vi "氨氮总氮总磷质控流程.vi"(8 "总氮":bool, 9 "总磷":bool, 10 "氨氮":bool, 11 "队列输入":refnum<queue>) -> (3 "布尔":bool)   [LabVIEW 2016, in "质控单元.lvlib"]
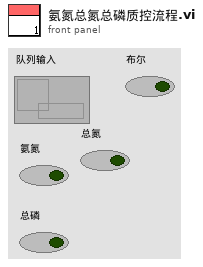
[diagram p1: front panel]
types:
  T1 = enum16{"待机", "启动氨氮水样", "氨氮测量中", "启动氨氮加标", "启动氨氮加标回收", "氨氮加标回收测量中", "启动总氮水样", "总氮测量中", "启动总氮加标", "启动总氮加标回收", "总氮加标回收测量中", "启动总磷水样", "总磷水样测量中", "启动总磷加标", "启动总磷加标回收", "总磷加标回收测量中", "结束"}
  T2 = cluster{"站号":u16, "量程切换":enum32{"H", "L", "AUTO"}, "控制命令":enum16{"启动测量", "标样核查", "零点核查", "跨度核查", "空白测试", "平行样测试", "加标回收", "空白校准", "标样校准", "初始化（清洗）", "停止测试", "仪器重启", "校时", "模式设置", "测量间隔设置"}, "模式设置":enum16{"待机", "连续模式", "周期模式", "定点模式", "受控模式", "手动模式"}, "测量间隔":u16}
  T3 = cluster{"时间标识":timestamp, "设备":string, "日志信息":string}
  T4 = cluster{"系统时间":timestamp, "工作状态":enum16{"空闲", "水样测试", "标样核查", "零点核查", "跨度核查", "空白测试", "平行样测试", "加标回收", "空白校准", "标样校准", "初始化（清洗）"}, "测量模式":enum16{"待机", "连续模式", "周期模式", "定点模式", "受控模式", "手动模式"}, "告警代码":enum16{"无告警", "缺试剂告警", "缺水样告警", "缺蒸馏水告警", "缺标液告警", "仪表漏液告警", "标定异常告警", "超量程告警", "加热异常", "低试剂预警", "超上限告警", "超下限告警", "仪表内部其他异常", "滴定异常告警", "电极异常告警", "量程切换告警", "参数设置告警", "PH电极电位异常", "电导率电极异常", "浊度光度异常", "溶解氧电极异常", "溶解氧光强异常", "温度异常告警", "PH异常告警", "溶解氧异常告警", "电导率异常告警", "浊度异常告警", "叶绿素异常告警", "藻密度异常告警", "蓝绿藻异常告警", "ORP异常告警", "氨氮异常告警", "清洁刷异常告警", "SD卡异常告警", "蓝牙异常告警", "Wifi异常告警", "流程异常告警"}, "故障代码":enum16{"无故障", "电机故障", "温度故障", "通讯故障", "滴定故障"}, "日志代码":u16, "软件版本":u16, "F0":sgl, "F1":sgl, "F2":sgl, "F3":sgl, "T":sgl, "H":sgl, "id":u16, "flowid":u16, "量程":u16}
  T5 = enum16{"空闲", "水样测试", "标样核查", "零点核查", "跨度核查", "空白测试", "平行样测试", "加标回收", "空白校准", "标样校准", "初始化（清洗）"}
  T6 = cluster{"因子编码":u32, "单位":u16, "标样参考值":sgl, "水样数据时间":timestamp, "水样实测值":sgl, "水样数据标识":string, "标样数据时间":timestamp, "标样实测值":sgl, "标样数据标识":string, "空白数据时间":timestamp, "空白实测值":sgl, "空白数据标识":string, "零点核查数据时间":timestamp, "零点核查实测值":sgl, "零点核查数据标识":string, "跨度核查数据时间":timestamp, "跨度核查实测值":sgl, "跨度核查数据标识":string, "加标回收数据时间":timestamp, "加标回收实测值":sgl, "加标回收数据标识":string, "平行样数据时间":timestamp, "平行样实测值":sgl, "平行样数据标识":string, "F0":sgl, "F1":sgl, "F2":sgl, "F3":sgl, "F4":sgl, "F5":sgl, "F6":sgl, "F7":sgl, "温度":sgl, "湿度":sgl, "X值":sgl}
  T7 = cluster{"量程":dbl, "检出限":dbl, "加标前水样浓度":dbl, "加标后水样浓度":dbl, "加标水杯定容体积":dbl, "加标母液浓度":dbl, "加标体积":dbl, "加标回收率":dbl}
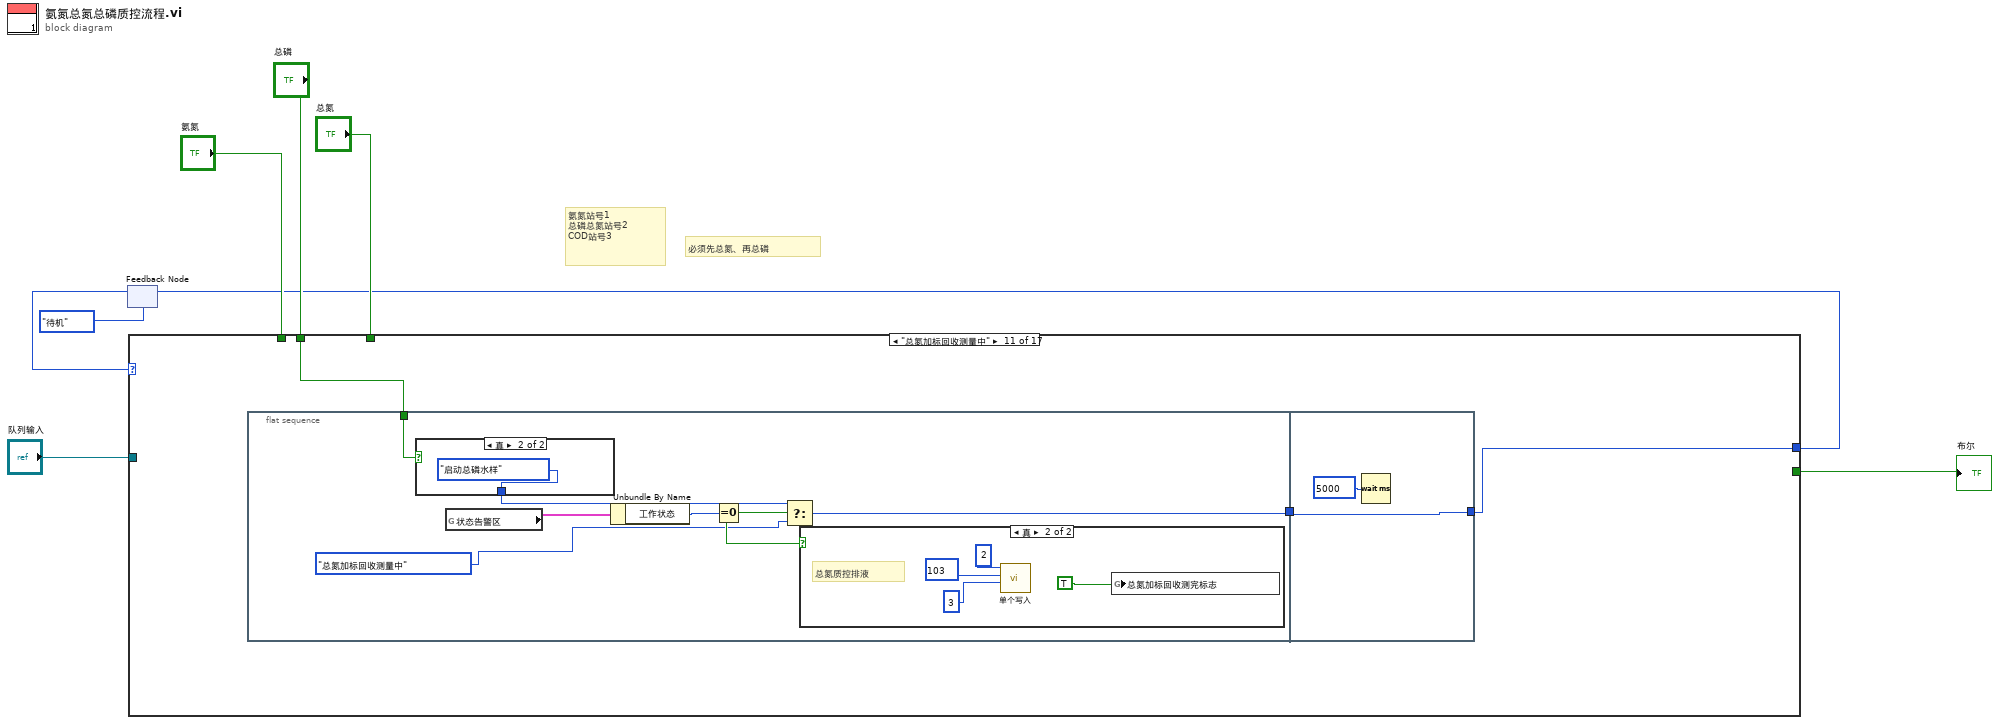
[diagram p0: block diagram]
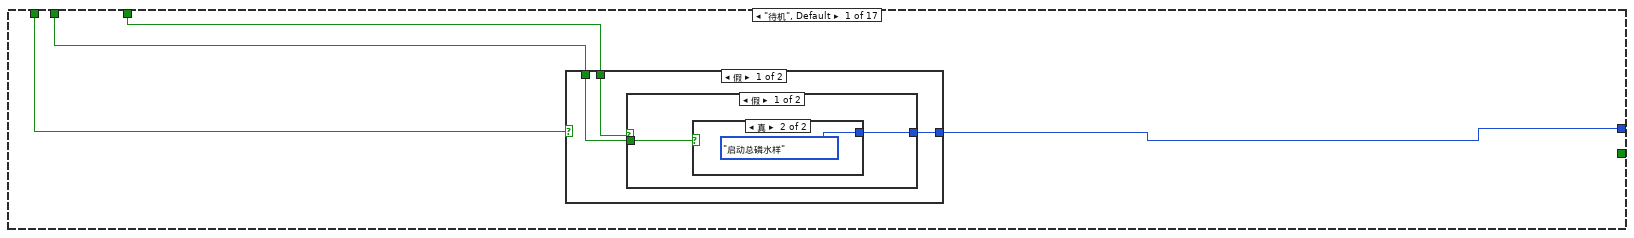
[diagram p2: hidden frame]
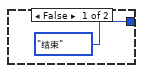
[diagram p3: hidden frame]
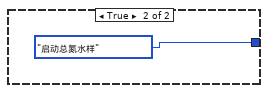
[diagram p4: hidden frame]
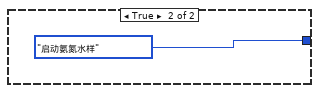
[diagram p5: hidden frame]
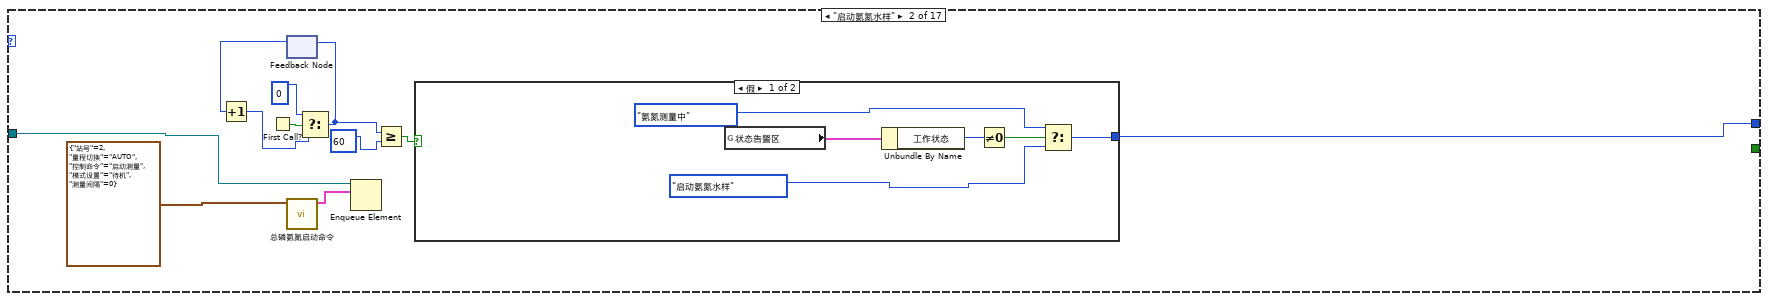
[diagram p6: hidden frame]
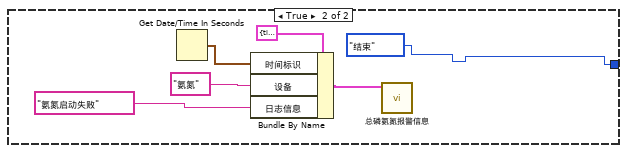
[diagram p7: hidden frame]
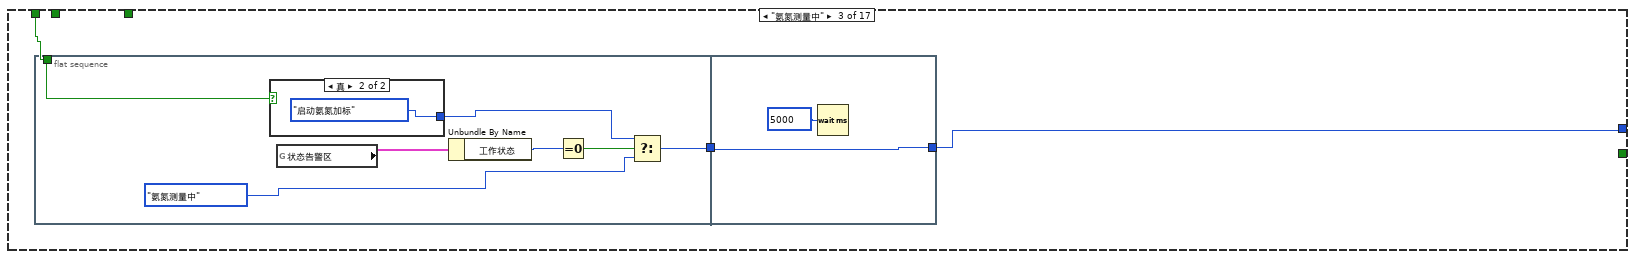
[diagram p8: hidden frame]
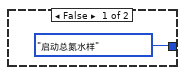
[diagram p9: hidden frame]
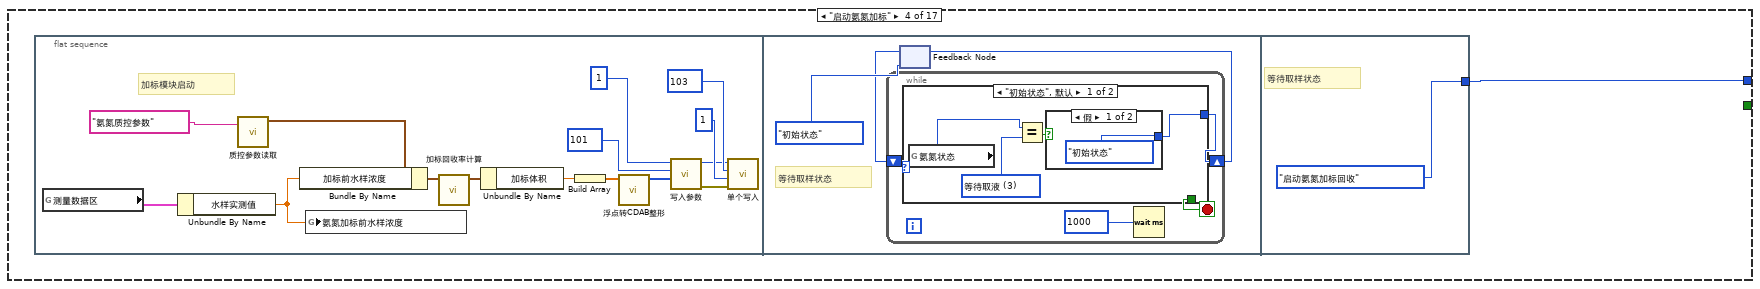
[diagram p10: hidden frame]
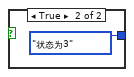
[diagram p11: hidden frame]
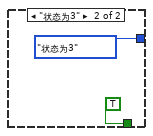
[diagram p12: hidden frame]
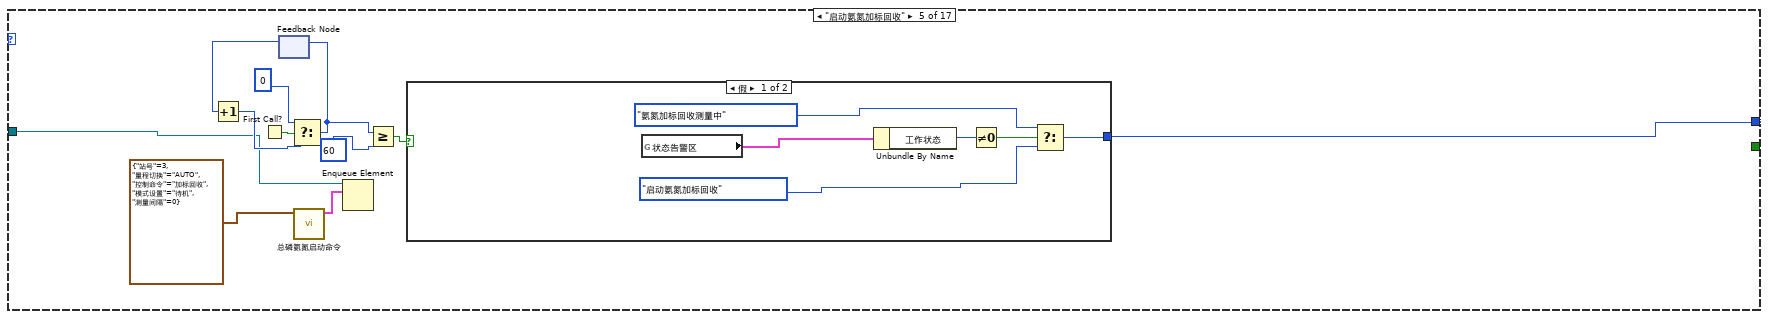
[diagram p13: hidden frame]
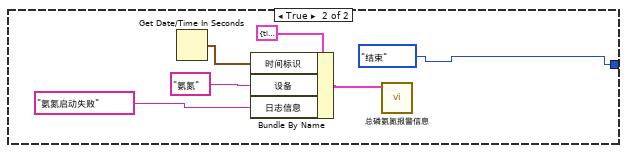
[diagram p14: hidden frame]
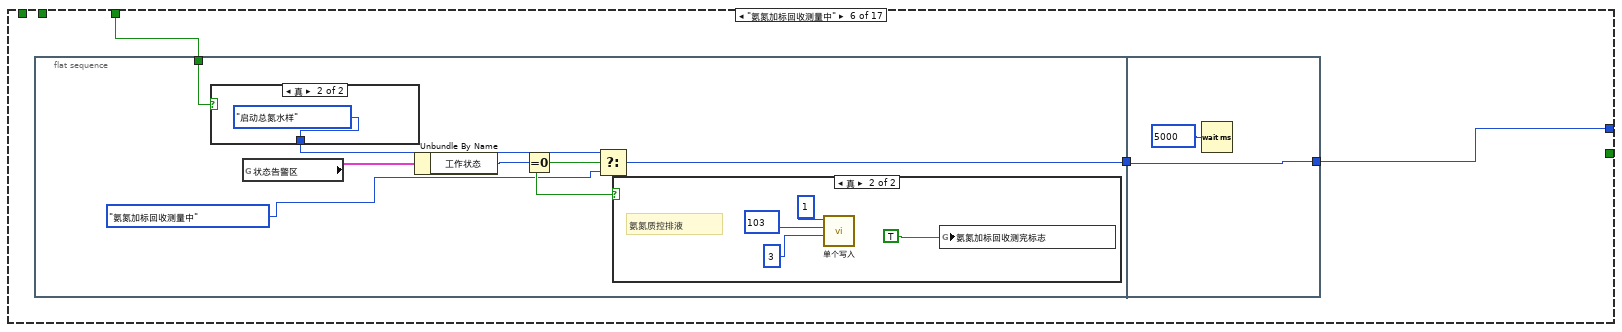
[diagram p15: hidden frame]
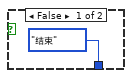
[diagram p16: hidden frame]
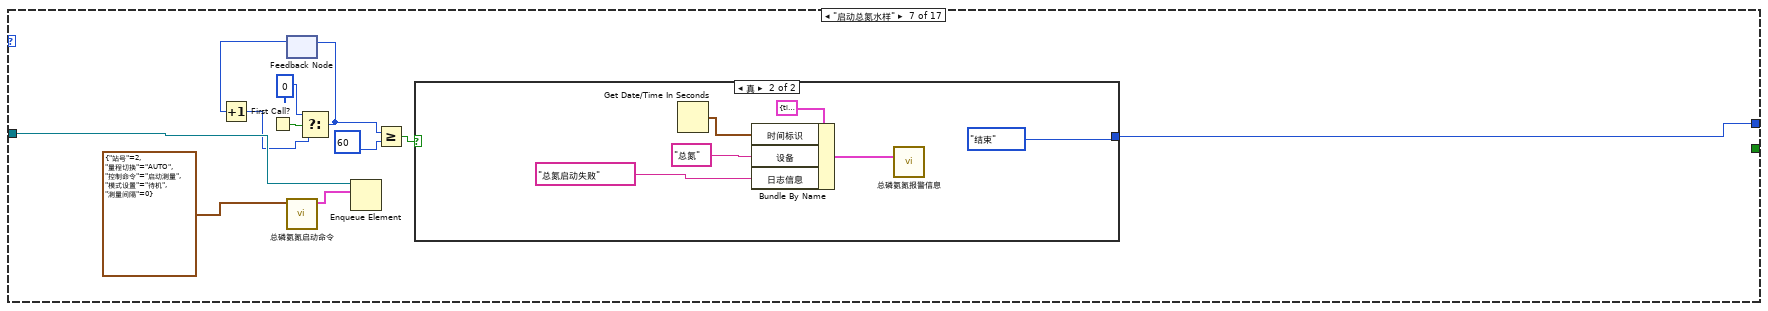
[diagram p18: hidden frame]
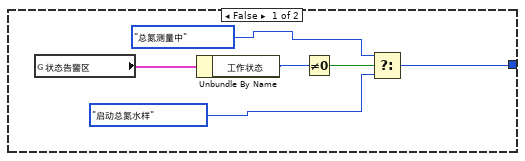
[diagram p19: hidden frame]
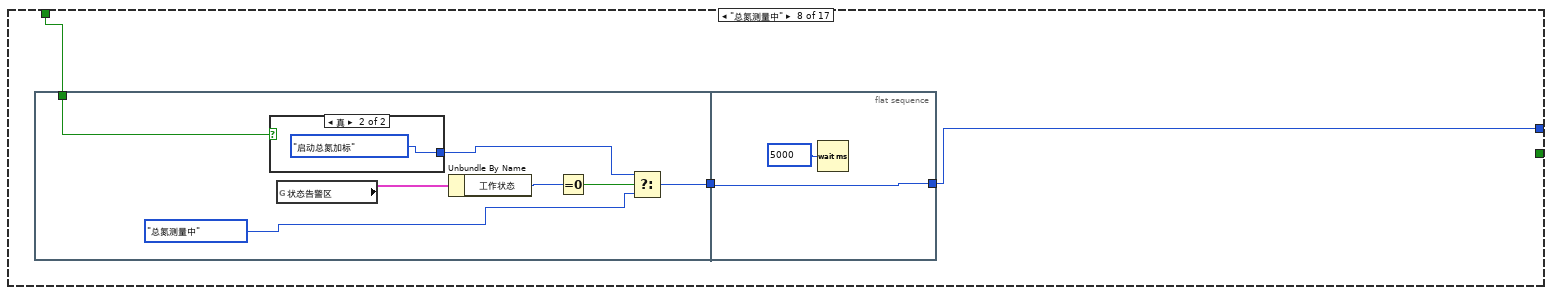
[diagram p20: hidden frame]
diagram:
  # "氨氮站号1   \n总磷总氮站号2\nCOD站号3"
  # "必须先总氮、再总磷"
  n1 = feedback #1(T1."待机") -> (w3:T1)
  n2 = case shown="\"总氮加标回收测量中\"" w3 {
    tunnel: [w12 w31 w47 w59 w92 w113 w140 w154 w168 w199 w222 w249 w265 w277 w309 w331 T1."结束"] -> w1
    tunnel: "队列输入" -> [_ w32 _ _ w93 _ w141 _ _ w202 _ w250 _ _ w310 _ _]
    tunnel: [_ _ _ _ _ _ _ _ _ _ _ _ _ _ _ _ TRUE] -> w6
    tunnel: "总磷" -> [w10 _ _ _ _ _ _ _ _ _ w223 _ w263 _ _ _ _]
    tunnel: "氨氮" -> [w11 _ w45 _ _ _ _ _ _ _ _ _ _ _ _ _ _]
    tunnel: "总氮" -> [w9 _ _ _ _ w114 _ w155 _ _ _ _ _ _ _ _ _]
    frame "待机", Default {
      n3 = case shown="假" w11 {
        tunnel: [w14 T1."启动氨氮水样"] -> w12
        tunnel: w10 -> [w15 _]
        tunnel: w9 -> [w13 _]
        frame False {
          n4 = case shown="假" w13 {
            tunnel: w15 -> [w16 _]
            tunnel: [w17 T1."启动总氮水样"] -> w14
            frame False {
              n5 = case shown="真" w16 {
                tunnel: [T1."结束" T1."启动总磷水样"] -> w17
                frame False {
                }
                frame True {
                }
              }
            }
            frame True {
            }
          }
        }
        frame True {
        }
      }
    }
    frame "启动氨氮水样" {
      n6 = First Call?() -> (First Call?: T/F=w29:bool)
      n7 = feedback #2() -> (w28:i32)  [unwired: 1 in]
      n8 = Increment(x=w28) -> (x+1=w27:i32)
      n9 = call "总磷氨氮启动命令.vi"("参数"=T2 {"站号"=2, "量程切换"=enum."AUTO", "控制命令"=enum."启动测量", "模式设置"=enum."待机", "测量间隔"=0}) -> ("启动命令"=w23:cluster{"命令":string, "data":variant})  [unwired: 10 in]
      n10 = Select(t=0, s=w29, f=w27) -> (s? t:f=w26:i32)
      n11 = feedback-in #2(w26) -> ()
      n12 = Enqueue Element(queue=w32, element=w23) -> ()  [unwired: 2 in, 3 out]
      n13 = Greater Or Equal?(x=w26, y=60) -> (x >= y?=w24:bool)
      n14 = case shown="假" w24 {
        tunnel: [w35 T1."结束"] -> w31
        frame False {
          n15 = global read "VAR总磷氨氮全局变量.vi" "状态告警区"() -> (w38:T4)
          n16 = Unbundle By Name(w38) -> ("工作状态"=w37:T5)
          n17 = Not Equal To 0?(x=w37) -> (x != 0?=w36:bool)
          n18 = Select(t=T1."氨氮测量中", s=w36, f=T1."启动氨氮水样") -> (s? t:f=w35:T1)
        }
        frame True {
          n19 = Get Date/Time In Seconds() -> (seconds since 1Jan1904=w44:timestamp)
          n20 = Bundle By Name(cluster=T3 {"时间标识"=timestamp(0 s since 1904-01-01), "设备"="", "日志信息"=""} ("data in"), "时间标识"=w44, "设备"="氨氮", "日志信息"="氨氮启动失败") -> (w40:T3)
          n21 = call "总磷氨氮报警信息.vi"("data in"=w40) -> ()  [unwired: 11 in]
        }
      }
    }
    frame "氨氮测量中" {
      n22 = flat-sequence {
        tunnel: [w52] -> w46
        tunnel: w45 -> [w49]
        tunnel: [w58] -> w47
        tunnel: w46 -> [w58]
        frame #0 {
          n23 = case shown="真" w49 {
            tunnel: [T1."启动总氮水样" T1."启动氨氮加标"] -> w50
            frame False {
            }
            frame True {
            }
          }
          n24 = global read "VAR总磷氨氮全局变量.vi" "状态告警区"() -> (w53:T4)
          n25 = Unbundle By Name(w53) -> ("工作状态"=w54:T5)
          n26 = Equal To 0?(x=w54) -> (x = 0?=w51:bool)
          n27 = Select(t=w50, s=w51, f=T1."氨氮测量中") -> (s? t:f=w52:T1)
        }
        frame #1 {
          n28 = Wait (ms)(milliseconds to wait=u32 5000 ("等待时间（毫秒）")) -> ()  [unwired: 1 out]
        }
      }
    }
    frame "启动氨氮加标" {
      n29 = flat-sequence {
        tunnel: [T1."启动氨氮加标回收"] -> w59
        frame #0 {
          w63 = u16 1 ("value")
          # "加标模块启动"
          n30 = global read "VAR总磷氨氮全局变量.vi" "测量数据区"() -> (w61:T6)
          n31 = Unbundle By Name(w61) -> ("水样实测值"=w60:sgl)
          n32 = call "质控参数读取.vi"("section"="氨氮质控参数") -> ("参数"=w71:T7)  [unwired: 9 in, 1 out]
          n33 = Bundle By Name(cluster=w71, "加标前水样浓度"=w60) -> (w72:T7)
          n34 = global write "水样浓度全局.vi" "氨氮加标前水样浓度"(w60) -> ()
          n35 = call "加标回收率计算.vi"("参数"=w72) -> ("参数 out"=w70:T7)  [unwired: 10 in]
          n36 = Unbundle By Name(w70) -> ("加标体积"=w62:dbl)
          n37 = Build Array(w62) -> (w69:dbl[])
          n38 = call "浮点转CDAB整形.vi"("浮点数"=w69) -> ("CDAB整形输出"=w64:u16[])  [unwired: 10 in]
          n39 = call "写入参数.vi"("values"=w64, "starting address"=u16 101, "Slave ID"=w63) -> ("error out"=w68:errorcluster)  [unwired: 8 in]
          n40 = call "单个写入.vi"("Error in"=w68, "value"=u16 1, "address"=u16 103, "Slave ID"=w63) -> ()  [unwired: 7 in, 1 out]
        }
        frame #1 {
          # "等待取样状态"
          n41 = feedback #3(enum16{"初始状态", "状态为3"}."初始状态") -> (w75:enum16{"初始状态", "状态为3"})
          n42 = while {
            shift-right: [w79] -> w74
            shift-left: w75 -> [w80]
            stop <- w78 stop-if-true
            n43 = case shown="\"初始状态\", 默认" w80 {
              tunnel: [w82 enum16{"初始状态", "状态为3"}."状态为3"] -> w79
              tunnel: [_ TRUE] -> w78
              frame "初始状态", Default {
                w81 = u16 3 items=["待机", "润洗", "进样", "等待取液", "排液"] ("氨氮状态")
                n44 = global read "氨氮加标回收状态全局变量.vi" "氨氮状态"() -> (w84:u16)
                n45 = Equal?(x=w84, y=w81) -> (x = y?=w83:bool)
                n46 = case shown="假" w83 {
                  tunnel: [enum16{"初始状态", "状态为3"}."初始状态" enum16{"初始状态", "状态为3"}."状态为3"] -> w82
                  frame False {
                  }
                  frame True {
                  }
                }
              }
              frame "状态为3" {
              }
            }
            n47 = Wait (ms)(milliseconds to wait=u32 1000 ("等待时间（毫秒）")) -> ()  [unwired: 1 out]
          }
          n48 = feedback-in #3(w74) -> ()
        }
        frame #2 {
          # "等待取样状态"
        }
      }
    }
    frame "启动氨氮加标回收" {
      n49 = First Call?() -> (First Call?: T/F=w99:bool)
      n50 = feedback #4() -> (w98:i32)  [unwired: 1 in]
      n51 = Increment(x=w98) -> (x+1=w97:i32)
      n52 = Select(t=0, s=w99, f=w97) -> (s? t:f=w96:i32)
      n53 = feedback-in #4(w96) -> ()
      n54 = call "总磷氨氮启动命令.vi"("参数"=T2 {"站号"=3, "量程切换"=enum."AUTO", "控制命令"=enum."加标回收", "模式设置"=enum."待机", "测量间隔"=0}) -> ("启动命令"=w91:cluster{"命令":string, "data":variant})  [unwired: 10 in]
      n55 = Enqueue Element(queue=w93, element=w91) -> ()  [unwired: 2 in, 3 out]
      n56 = Greater Or Equal?(x=w96, y=60) -> (x >= y?=w94:bool)
      n57 = case shown="假" w94 {
        tunnel: [w103 T1."结束"] -> w92
        frame False {
          n58 = global read "VAR总磷氨氮全局变量.vi" "状态告警区"() -> (w106:T4)
          n59 = Unbundle By Name(w106) -> ("工作状态"=w105:T5)
          n60 = Not Equal To 0?(x=w105) -> (x != 0?=w104:bool)
          n61 = Select(t=T1."氨氮加标回收测量中", s=w104, f=T1."启动氨氮加标回收") -> (s? t:f=w103:T1)
        }
        frame True {
          n62 = Get Date/Time In Seconds() -> (seconds since 1Jan1904=w112:timestamp)
          n63 = Bundle By Name(cluster=T3 {"时间标识"=timestamp(0 s since 1904-01-01), "设备"="", "日志信息"=""} ("data in"), "时间标识"=w112, "设备"="氨氮", "日志信息"="氨氮启动失败") -> (w108:T3)
          n64 = call "总磷氨氮报警信息.vi"("data in"=w108) -> ()  [unwired: 11 in]
        }
      }
    }
    frame "氨氮加标回收测量中" {
      n65 = flat-sequence {
        tunnel: [w120] -> w115
        tunnel: w114 -> [w117]
        tunnel: [w130] -> w113
        tunnel: w115 -> [w130]
        frame #0 {
          n66 = case shown="真" w117 {
            tunnel: [T1."结束" T1."启动总氮水样"] -> w119
            frame False {
            }
            frame True {
            }
          }
          n67 = global read "VAR总磷氨氮全局变量.vi" "状态告警区"() -> (w121:T4)
          n68 = Unbundle By Name(w121) -> ("工作状态"=w122:T5)
          n69 = Equal To 0?(x=w122) -> (x = 0?=w118:bool)
          n70 = Select(t=w119, s=w118, f=T1."氨氮加标回收测量中") -> (s? t:f=w120:T1)
          n71 = case shown="真" w118 {
            frame False {
            }
            frame True {
              # "氨氮质控排液"
              n72 = call "单个写入.vi"("value"=u16 3, "address"=u16 103, "Slave ID"=u8 1) -> ()  [unwired: 8 in, 1 out]
              n73 = global write "质控测完标志全局 1.vi" "氨氮加标回收测完标志"(TRUE) -> ()
            }
          }
        }
        frame #1 {
          n74 = Wait (ms)(milliseconds to wait=u32 5000 ("等待时间（毫秒）")) -> ()  [unwired: 1 out]
        }
      }
    }
    frame "启动总氮水样" {
      n75 = First Call?() -> (First Call?: T/F=w138:bool)
      n76 = feedback #5() -> (w137:i32)  [unwired: 1 in]
      n77 = Increment(x=w137) -> (x+1=w136:i32)
      n78 = call "总磷氨氮启动命令.vi"("参数"=T2 {"站号"=2, "量程切换"=enum."AUTO", "控制命令"=enum."启动测量", "模式设置"=enum."待机", "测量间隔"=0}) -> ("启动命令"=w132:cluster{"命令":string, "data":variant})  [unwired: 10 in]
      n79 = Select(t=0, s=w138, f=w136) -> (s? t:f=w135:i32)
      n80 = feedback-in #5(w135) -> ()
      n81 = Enqueue Element(queue=w141, element=w132) -> ()  [unwired: 2 in, 3 out]
      n82 = Greater Or Equal?(x=w135, y=60) -> (x >= y?=w133:bool)
      n83 = case shown="真" w133 {
        tunnel: [w144 T1."结束"] -> w140
        frame False {
          n84 = global read "VAR总磷氨氮全局变量.vi" "状态告警区"() -> (w145:T4)
          n85 = Unbundle By Name(w145) -> ("工作状态"=w146:T5)
          n86 = Not Equal To 0?(x=w146) -> (x != 0?=w147:bool)
          n87 = Select(t=T1."总氮测量中", s=w147, f=T1."启动总氮水样") -> (s? t:f=w144:T1)
        }
        frame True {
          n88 = Get Date/Time In Seconds() -> (seconds since 1Jan1904=w153:timestamp)
          n89 = Bundle By Name(cluster=T3 {"时间标识"=timestamp(0 s since 1904-01-01), "设备"="", "日志信息"=""} ("data in"), "时间标识"=w153, "设备"="总氮", "日志信息"="总氮启动失败") -> (w149:T3)
          n90 = call "总磷氨氮报警信息.vi"("data in"=w149) -> ()  [unwired: 11 in]
        }
      }
    }
    frame "总氮测量中" {
      n91 = flat-sequence {
        tunnel: [w161] -> w156
        tunnel: w155 -> [w158]
        tunnel: [w167] -> w154
        tunnel: w156 -> [w167]
        frame #0 {
          n92 = case shown="真" w158 {
            tunnel: [T1."启动总磷水样" T1."启动总氮加标"] -> w159
            frame False {
            }
            frame True {
            }
          }
          n93 = global read "VAR总磷氨氮全局变量.vi" "状态告警区"() -> (w162:T4)
          n94 = Unbundle By Name(w162) -> ("工作状态"=w163:T5)
          n95 = Equal To 0?(x=w163) -> (x = 0?=w160:bool)
          n96 = Select(t=w159, s=w160, f=T1."总氮测量中") -> (s? t:f=w161:T1)
        }
        frame #1 {
          n97 = Wait (ms)(milliseconds to wait=u32 5000 ("等待时间（毫秒）")) -> ()  [unwired: 1 out]
        }
      }
    }
    frame "启动总氮加标" {
      n98 = flat-sequence {
        tunnel: [T1."启动总氮加标回收"] -> w168
        frame #0 {
          w173 = u16 2 ("value")
          # "加标模块启动"
          n99 = global read "VAR总磷氨氮全局变量.vi" "测量数据区"() -> (w171:T6)
          n100 = Unbundle By Name(w171) -> ("水样实测值"=w169:sgl)
          n101 = call "质控参数读取.vi"("section"="总氮质控参数") -> ("参数"=w170:T7)  [unwired: 9 in, 1 out]
          n102 = Bundle By Name(cluster=w170, "加标前水样浓度"=w169) -> (w181:T7)
          n103 = global write "水样浓度全局.vi" "总氮加标前水样浓度"(w169) -> ()
          n104 = call "加标回收率计算.vi"("参数"=w181) -> ("参数 out"=w180:T7)  [unwired: 10 in]
          n105 = Unbundle By Name(w180) -> ("加标体积"=w172:dbl)
          n106 = Build Array(w172) -> (w179:dbl[])
          n107 = call "浮点转CDAB整形.vi"("浮点数"=w179) -> ("CDAB整形输出"=w174:u16[])  [unwired: 10 in]
          n108 = call "写入参数.vi"("values"=w174, "starting address"=u16 101, "Slave ID"=w173) -> ("error out"=w178:errorcluster)  [unwired: 8 in]
          n109 = call "单个写入.vi"("Error in"=w178, "value"=u16 2, "address"=u16 103, "Slave ID"=w173) -> ()  [unwired: 7 in, 1 out]
        }
        frame #1 {
          # "等待取样状态"
          n110 = feedback #6(enum16{"初始状态", "状态为3"}."初始状态") -> (w184:enum16{"初始状态", "状态为3"})
          n111 = while {
            shift-right: [w188] -> w183
            shift-left: w184 -> [w189]
            stop <- w187 stop-if-true
            n112 = case shown="\"状态为3\"" w189 {
              tunnel: [w190 enum16{"初始状态", "状态为3"}."状态为3"] -> w188
              tunnel: [_ TRUE] -> w187
              frame "初始状态", Default {
                n113 = global read "氨氮加标回收状态全局变量.vi" "总磷状态"() -> (w192:u16)
                n114 = Equal?(x=w192, y=u16 3) -> (x = y?=w191:bool)
                n115 = case shown="真" w191 {
                  tunnel: [enum16{"初始状态", "状态为3"}."初始状态" enum16{"初始状态", "状态为3"}."状态为3"] -> w190
                  frame False {
                  }
                  frame True {
                  }
                }
              }
              frame "状态为3" {
              }
            }
            n116 = Wait (ms)(milliseconds to wait=u32 1000 ("等待时间（毫秒）")) -> ()  [unwired: 1 out]
          }
          n117 = feedback-in #6(w183) -> ()
        }
        frame #2 {
          # "等待取样状态"
        }
      }
    }
    frame "启动总氮加标回收" {
      n118 = First Call?() -> (First Call?: T/F=w208:bool)
      n119 = feedback #7() -> (w207:i32)  [unwired: 1 in]
      n120 = Increment(x=w207) -> (x+1=w206:i32)
      n121 = call "总磷氨氮启动命令.vi"("参数"=T2 {"站号"=2, "量程切换"=enum."AUTO", "控制命令"=enum."加标回收", "模式设置"=enum."待机", "测量间隔"=0}) -> ("启动命令"=w200:cluster{"命令":string, "data":variant})  [unwired: 10 in]
      n122 = Select(t=0, s=w208, f=w206) -> (s? t:f=w205:i32)
      n123 = feedback-in #7(w205) -> ()
      n124 = Enqueue Element(queue=w202, element=w200) -> ()  [unwired: 2 in, 3 out]
      n125 = Greater Or Equal?(x=w205, y=60) -> (x >= y?=w203:bool)
      n126 = case shown="假" w203 {
        tunnel: [w212 T1."结束"] -> w199
        frame False {
          n127 = global read "VAR总磷氨氮全局变量.vi" "状态告警区"() -> (w215:T4)
          n128 = Unbundle By Name(w215) -> ("工作状态"=w214:T5)
          n129 = Not Equal To 0?(x=w214) -> (x != 0?=w213:bool)
          n130 = Select(t=T1."总氮加标回收测量中", s=w213, f=T1."启动总氮加标回收") -> (s? t:f=w212:T1)
        }
        frame True {
          n131 = Get Date/Time In Seconds() -> (seconds since 1Jan1904=w221:timestamp)
          n132 = Bundle By Name(cluster=T3 {"时间标识"=timestamp(0 s since 1904-01-01), "设备"="", "日志信息"=""} ("data in"), "时间标识"=w221, "设备"="氨氮", "日志信息"="氨氮启动失败") -> (w217:T3)
          n133 = call "总磷氨氮报警信息.vi"("data in"=w217) -> ()  [unwired: 11 in]
        }
      }
    }
    frame "总氮加标回收测量中" {
      n134 = flat-sequence {
        tunnel: [w229] -> w224
        tunnel: w223 -> [w226]
        tunnel: [w239] -> w222
        tunnel: w224 -> [w239]
        frame #0 {
          n135 = case shown="真" w226 {
            tunnel: [T1."结束" T1."启动总磷水样"] -> w228
            frame False {
            }
            frame True {
            }
          }
          n136 = global read "VAR总磷氨氮全局变量.vi" "状态告警区"() -> (w230:T4)
          n137 = Unbundle By Name(w230) -> ("工作状态"=w231:T5)
          n138 = Equal To 0?(x=w231) -> (x = 0?=w227:bool)
          n139 = Select(t=w228, s=w227, f=T1."总氮加标回收测量中") -> (s? t:f=w229:T1)
          n140 = case shown="真" w227 {
            frame False {
            }
            frame True {
              # "总氮质控排液"
              n141 = call "单个写入.vi"("value"=u16 3, "address"=u16 103, "Slave ID"=u8 2) -> ()  [unwired: 8 in, 1 out]
              n142 = global write "质控测完标志全局 1.vi" "总氮加标回收测完标志"(TRUE) -> ()
            }
          }
        }
        frame #1 {
          n143 = Wait (ms)(milliseconds to wait=u32 5000 ("等待时间（毫秒）")) -> ()  [unwired: 1 out]
        }
      }
    }
    frame "启动总磷水样" {
      n144 = First Call?() -> (First Call?: T/F=w247:bool)
      n145 = feedback #8() -> (w246:i32)  [unwired: 1 in]
      n146 = Increment(x=w246) -> (x+1=w245:i32)
      n147 = call "总磷氨氮启动命令.vi"("参数"=T2 {"站号"=1, "量程切换"=enum."AUTO", "控制命令"=enum."启动测量", "模式设置"=enum."待机", "测量间隔"=0}) -> ("启动命令"=w241:cluster{"命令":string, "data":variant})  [unwired: 10 in]
      n148 = Select(t=0, s=w247, f=w245) -> (s? t:f=w244:i32)
      n149 = feedback-in #8(w244) -> ()
      n150 = Enqueue Element(queue=w250, element=w241) -> ()  [unwired: 2 in, 3 out]
      n151 = Greater Or Equal?(x=w244, y=60) -> (x >= y?=w242:bool)
      n152 = case shown="假" w242 {
        tunnel: [w253 T1."结束"] -> w249
        frame False {
          n153 = global read "VAR总磷氨氮全局变量.vi" "状态告警区"() -> (w254:T4)
          n154 = Unbundle By Name(w254) -> ("工作状态"=w255:T5)
          n155 = Not Equal To 0?(x=w255) -> (x != 0?=w256:bool)
          n156 = Select(t=T1."总磷水样测量中", s=w256, f=T1."启动总磷水样") -> (s? t:f=w253:T1)
        }
        frame True {
          n157 = Get Date/Time In Seconds() -> (seconds since 1Jan1904=w262:timestamp)
          n158 = Bundle By Name(cluster=T3 {"时间标识"=timestamp(0 s since 1904-01-01), "设备"="", "日志信息"=""} ("data in"), "时间标识"=w262, "设备"="总磷", "日志信息"="总磷启动失败") -> (w258:T3)
          n159 = call "总磷氨氮报警信息.vi"("data in"=w258) -> ()  [unwired: 11 in]
        }
      }
    }
    frame "总磷水样测量中" {
      n160 = flat-sequence {
        tunnel: [w270] -> w264
        tunnel: w263 -> [w267]
        tunnel: [w276] -> w265
        tunnel: w264 -> [w276]
        frame #0 {
          n161 = case shown="真" w267 {
            tunnel: [T1."结束" T1."启动总磷加标"] -> w268
            frame False {
            }
            frame True {
            }
          }
          n162 = global read "VAR总磷氨氮全局变量.vi" "状态告警区"() -> (w271:T4)
          n163 = Unbundle By Name(w271) -> ("工作状态"=w272:T5)
          n164 = Equal To 0?(x=w272) -> (x = 0?=w269:bool)
          n165 = Select(t=w268, s=w269, f=T1."总磷水样测量中") -> (s? t:f=w270:T1)
        }
        frame #1 {
          n166 = Wait (ms)(milliseconds to wait=u32 5000 ("等待时间（毫秒）")) -> ()  [unwired: 1 out]
        }
      }
    }
    frame "启动总磷加标" {
      n167 = flat-sequence {
        tunnel: [T1."启动总磷加标回收"] -> w277
        frame #0 {
          w282 = u16 2 ("value")
          # "加标模块启动"
          n168 = global read "VAR总磷氨氮全局变量.vi" "测量数据区"() -> (w280:T6)
          n169 = Unbundle By Name(w280) -> ("水样实测值"=w278:sgl)
          n170 = call "质控参数读取.vi"("section"="总磷质控参数") -> ("参数"=w279:T7)  [unwired: 9 in, 1 out]
          n171 = Bundle By Name(cluster=w279, "加标前水样浓度"=w278) -> (w290:T7)
          n172 = global write "水样浓度全局.vi" "总磷加标前水样浓度"(w278) -> ()
          n173 = call "加标回收率计算.vi"("参数"=w290) -> ("参数 out"=w289:T7)  [unwired: 10 in]
          n174 = Unbundle By Name(w289) -> ("加标体积"=w281:dbl)
          n175 = Build Array(w281) -> (w288:dbl[])
          n176 = call "浮点转CDAB整形.vi"("浮点数"=w288) -> ("CDAB整形输出"=w283:u16[])  [unwired: 10 in]
          n177 = call "写入参数.vi"("values"=w283, "starting address"=u16 101, "Slave ID"=w282) -> ("error out"=w287:errorcluster)  [unwired: 8 in]
          n178 = call "单个写入.vi"("Error in"=w287, "value"=u16 2, "address"=u16 103, "Slave ID"=w282) -> ()  [unwired: 7 in, 1 out]
        }
        frame #1 {
          # "等待取样状态"
          n179 = feedback #9(enum16{"初始状态", "状态为3"}."初始状态") -> (w293:enum16{"初始状态", "状态为3"})
          n180 = while {
            shift-right: [w297] -> w292
            shift-left: w293 -> [w298]
            stop <- w296 stop-if-true
            n181 = case shown="\"状态为3\"" w298 {
              tunnel: [w299 enum16{"初始状态", "状态为3"}."状态为3"] -> w297
              tunnel: [_ TRUE] -> w296
              frame "初始状态", Default {
                n182 = global read "氨氮加标回收状态全局变量.vi" "总磷状态"() -> (w301:u16)
                n183 = Equal?(x=w301, y=u16 3) -> (x = y?=w300:bool)
                n184 = case shown="真" w300 {
                  tunnel: [enum16{"初始状态", "状态为3"}."初始状态" enum16{"初始状态", "状态为3"}."状态为3"] -> w299
                  frame False {
                  }
                  frame True {
                  }
                }
              }
              frame "状态为3" {
              }
            }
            n185 = Wait (ms)(milliseconds to wait=u32 1000 ("等待时间（毫秒）")) -> ()  [unwired: 1 out]
          }
          n186 = feedback-in #9(w292) -> ()
        }
        frame #2 {
          # "等待取样状态"
        }
      }
    }
    frame "启动总磷加标回收" {
      n187 = First Call?() -> (First Call?: T/F=w317:bool)
      n188 = feedback #10() -> (w316:i32)  [unwired: 1 in]
      n189 = Increment(x=w316) -> (x+1=w315:i32)
      n190 = call "总磷氨氮启动命令.vi"("参数"=T2 {"站号"=1, "量程切换"=enum."AUTO", "控制命令"=enum."加标回收", "模式设置"=enum."待机", "测量间隔"=0}) -> ("启动命令"=w311:cluster{"命令":string, "data":variant})  [unwired: 10 in]
      n191 = Select(t=0, s=w317, f=w315) -> (s? t:f=w314:i32)
      n192 = feedback-in #10(w314) -> ()
      n193 = Enqueue Element(queue=w310, element=w311) -> ()  [unwired: 2 in, 3 out]
      n194 = Greater Or Equal?(x=w314, y=60) -> (x >= y?=w312:bool)
      n195 = case shown="真" w312 {
        tunnel: [w321 T1."结束"] -> w309
        frame False {
          n196 = global read "VAR总磷氨氮全局变量.vi" "状态告警区"() -> (w322:T4)
          n197 = Unbundle By Name(w322) -> ("工作状态"=w323:T5)
          n198 = Not Equal To 0?(x=w323) -> (x != 0?=w324:bool)
          n199 = Select(t=T1."总磷加标回收测量中", s=w324, f=T1."启动总磷加标回收") -> (s? t:f=w321:T1)
        }
        frame True {
          n200 = Get Date/Time In Seconds() -> (seconds since 1Jan1904=w330:timestamp)
          n201 = Bundle By Name(cluster=T3 {"时间标识"=timestamp(0 s since 1904-01-01), "设备"="", "日志信息"=""} ("data in"), "时间标识"=w330, "设备"="总磷", "日志信息"="总磷启动失败") -> (w326:T3)
          n202 = call "总磷氨氮报警信息.vi"("data in"=w326) -> ()  [unwired: 11 in]
        }
      }
    }
    frame "总磷加标回收测量中" {
      n203 = flat-sequence {
        tunnel: [w336] -> w332
        tunnel: [w344] -> w331
        tunnel: w332 -> [w344]
        frame #0 {
          n204 = global read "VAR总磷氨氮全局变量.vi" "状态告警区"() -> (w337:T4)
          n205 = Unbundle By Name(w337) -> ("工作状态"=w338:T5)
          n206 = Equal To 0?(x=w338) -> (x = 0?=w335:bool)
          n207 = Select(t=T1."结束", s=w335, f=T1."总磷加标回收测量中") -> (s? t:f=w336:T1)
          n208 = case shown="真" w335 {
            frame False {
            }
            frame True {
              # "总磷质控排液"
              n209 = global write "质控测完标志全局 1.vi" "总磷加标回收测完标志"(TRUE) -> ()
              n210 = call "单个写入.vi"("value"=u16 3, "address"=u16 103, "Slave ID"=u8 2) -> ()  [unwired: 8 in, 1 out]
            }
          }
        }
        frame #1 {
          n211 = Wait (ms)(milliseconds to wait=u32 5000 ("等待时间（毫秒）")) -> ()  [unwired: 1 out]
        }
      }
    }
    frame "结束" {
    }
  }
  "布尔" <- w6
  n212 = feedback-in #1(w1) -> ()
